vi "Error Handler SubLoops.vi"(8 "error in":errorcluster, 11 "main gui queue":refnum<queue>) -> (0 "error out":errorcluster)   [LabVIEW 2020]
uses:
  GUI/Main GUI Loop/Handler.ctl
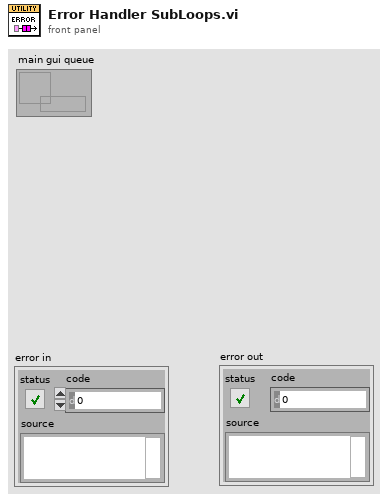
[diagram p1: front panel]
types:
  T1 = typedef "Handler.ctl" = cluster{"bool ref":refnum<vi>, "error":errorcluster, "msg":string, "status":string, "switch status":bool}
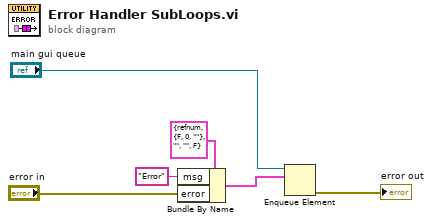
[diagram p0: block diagram]
diagram:
  n1 = Bundle By Name(cluster=T1 {"bool ref"=refnum, "error"={"status"=FALSE, "code"=0, "source"=""}, "msg"="", "status"="", "switch status"=FALSE} ("main gui"), "msg"="Error", "error"="error in") -> (w4:T1)
  n2 = Enqueue Element(queue="main gui queue", element=w4) -> (error out=→"error out":errorcluster)  [unwired: 2 in, 2 out]
